vi "Lancador1.vi"() -> ()   [LabVIEW 2019]
panel:
  out "lancadorA":dbl
  out "Lancador1":dbl
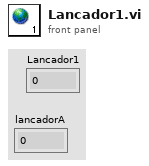
[diagram p1: front panel]
diagram:
